vi "Get Character Map.vi"() -> (2 "Symbol Map (Small Fonts 8)":map{string, T1}(c390))   [LabVIEW 2021, in "Picture Pixel Fonts.lvlib" / "Pixel Font.lvlib"]
uses:
  Pixel Font.lvlib
  <vilib>/picture/picture.llb/imagedata.ctl
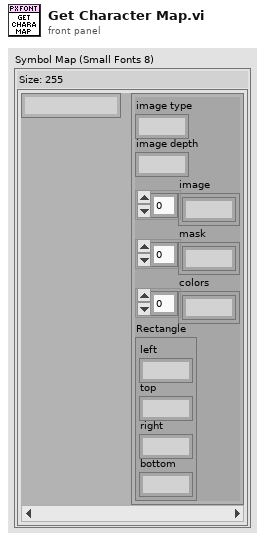
[diagram p1: front panel]
types:
  T1 = typedef "imagedata.ctl" = cluster{"image type":i32, "image depth":i32, "image":u8[], "mask":u8[], "colors":u32[], "Rectangle":cluster{"left":i16, "top":i16, "right":i16, "bottom":i16}}
  T2 = cluster{"horizontal":enum16{"left", "center", "right"}, "vertical":enum16{"top", "center", "bottom"}}
  T3 = enum16{"User-specified Font", "Application Font", "System Font", "Dialog Font"}
  T4 = cluster{"Font Name:":string, "Size":i16, "Strikeout?":bool, "Italic?":bool, "Underline?":bool, "Outline?":bool, "Shadow?":bool, "Bold?":bool}
  T5 = enum16{"None", "Stacked", "Clockwise", "Counterclockwise"}
  T6 = cluster{"left":i16, "top":i16, "right":i16, "bottom":i16}
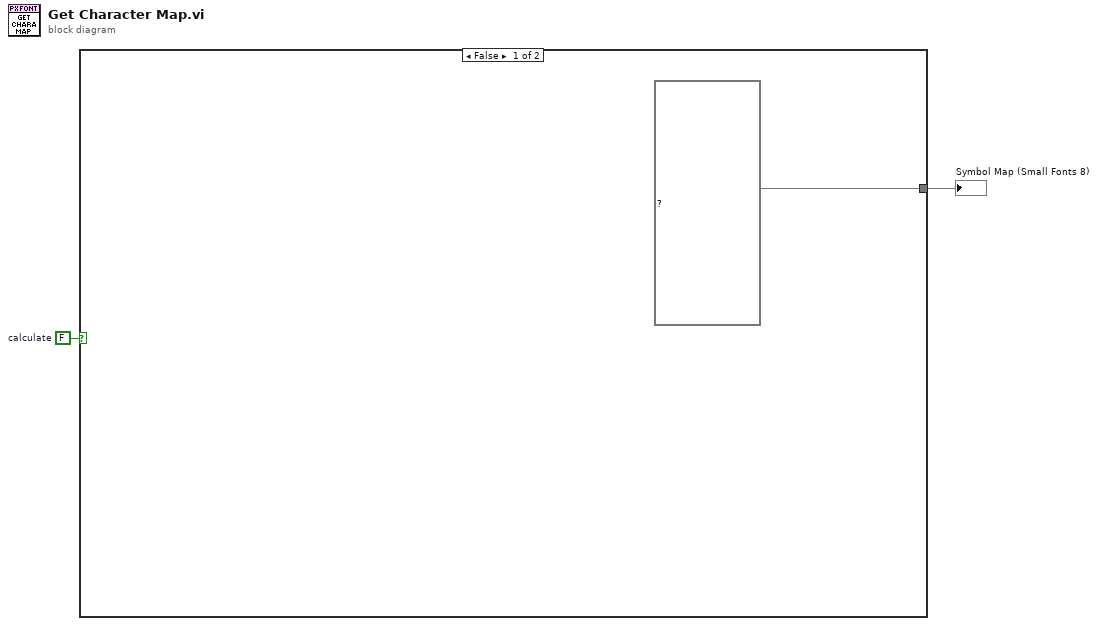
[diagram p0: block diagram]
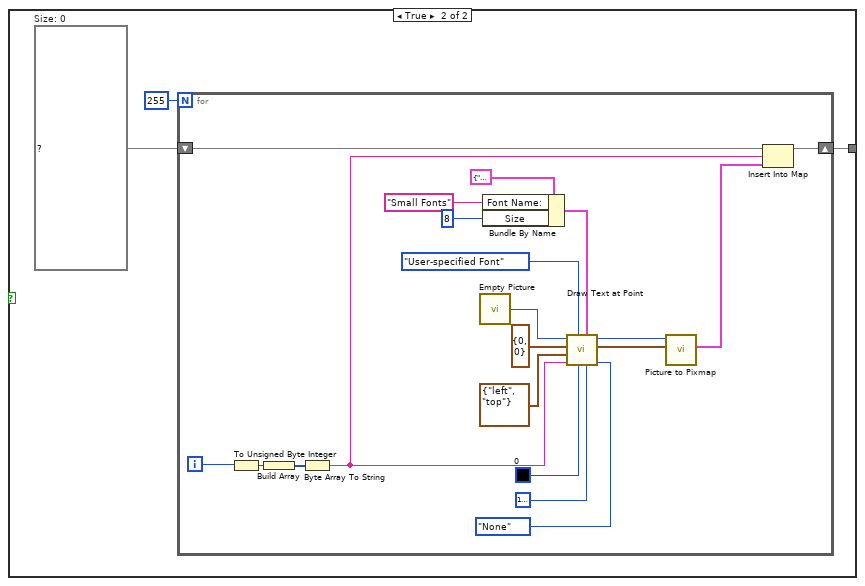
[diagram p2: hidden frame]
diagram:
  w1 = FALSE  # calculate
  n1 = case shown="False" w1 {
    tunnel: [map{string, T1} data[29515B] ("Symbol Map (Small Fonts 8)") w4] -> w2
    frame False {
    }
    frame True {
      w5 = map{string, T1} {}  # Size: 0
      n2 = for {
        N: 255 -> [_]
        shift-right: [w15] -> w4
        shift-left: w5 -> [w16]
        i -> [w14]
        n3 = To Unsigned Byte Integer(number=w14) -> (unsigned 8bit integer=w12:u8)
        n4 = Build Array(w12) -> (w13:u8[])
        n5 = Byte Array To String(unsigned byte array=w13) -> (string=w11:string)
        n6 = call "Empty Picture"() -> ("empty picture"=w9:picture)
        n7 = Bundle By Name(cluster=T4 {"Font Name:"="", "Size"=0, "Strikeout?"=FALSE, "Italic?"=FALSE, "Underline?"=FALSE, "Outline?"=FALSE, "Shadow?"=FALSE, "Bold?"=FALSE} ("[user-specified font]"), "Font Name:"="Small Fonts", "Size"=i16 8) -> (w19:T4)
        n8 = call <vilib>:"Draw Text at Point.vi"("text orientation"=T5."None", "BG color(transparent)"=u32 16777216, "[user-specified font]"=w19, "text color(black)"=u32 0, "desired font(Application)"=T3."User-specified Font", "text"=w11, "alignment(left, top)"=T2 {"horizontal"=enum."left", "vertical"=enum."top"}, "origin"=cluster{"x":i16, "y":i16} {"x"=0, "y"=0}, "picture"=w9) -> ("text rect"=w8:T6, "new picture"=w20:picture)  [unwired: 1 out]
        n9 = call <vilib>:"Picture to Pixmap.vi"("rect"=w8, "picture"=w20) -> ("image data"=w10:T1)  [unwired: 8 in, 1 out]
        n10 = Insert Into Map(map in=w16, key=w11, value=w10) -> (map out=w15:map{string, T1})  [unwired: 2 out]
      }
    }
  }
  "Symbol Map (Small Fonts 8)" <- w2
